vi "Testing Trigger.vi"() -> ()   [LabVIEW 2022 SP3]
panel:
  in  "2400 GPIB add":string="24"
  in  "2182 GPIB add":string="25"
  out "Delta Readings (uV)":ext[](array[numeric]) format="%.12f"
  out "Voltage Drop Across DUT":dbl[](graph)
  in  "Sample Count To Display":i32=10
  out "Resistance (m-Ohms)":dbl[](array[numeric]) format="%.10f"
  out "Resistance of DUT":dbl[](graph)
  in  "2400 Trig Count":string="20"
  in  "2182 Buffer Points":string="10"
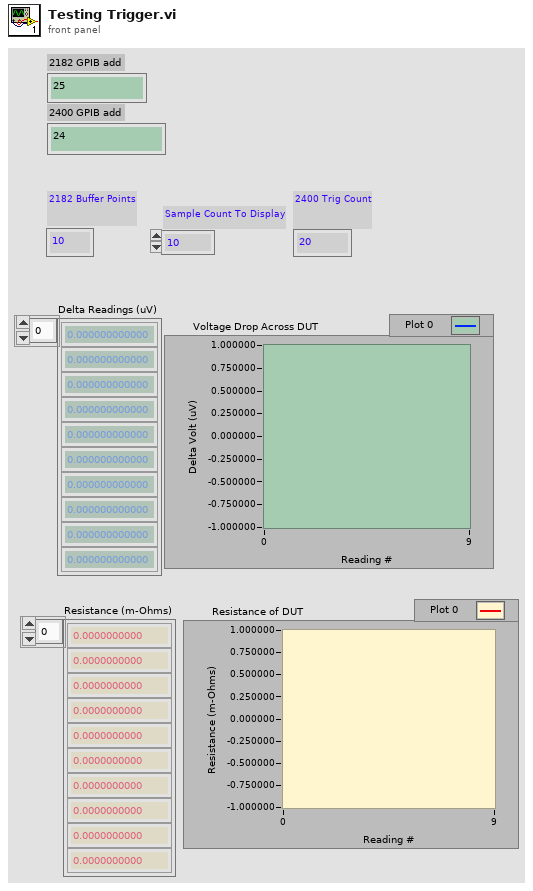
[diagram p1: front panel]
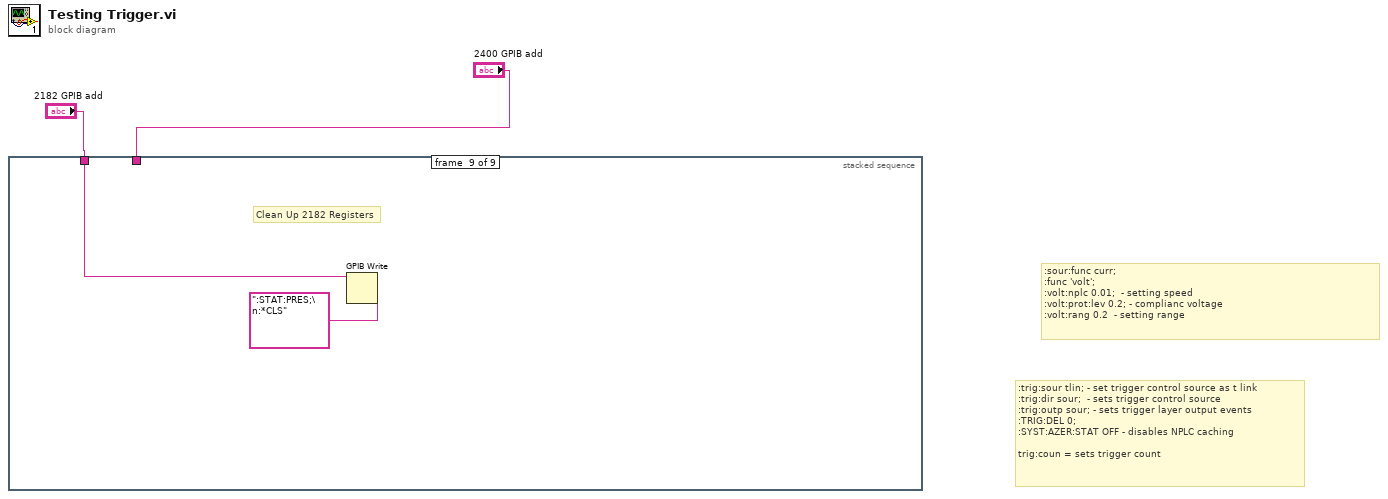
[diagram p0: block diagram]
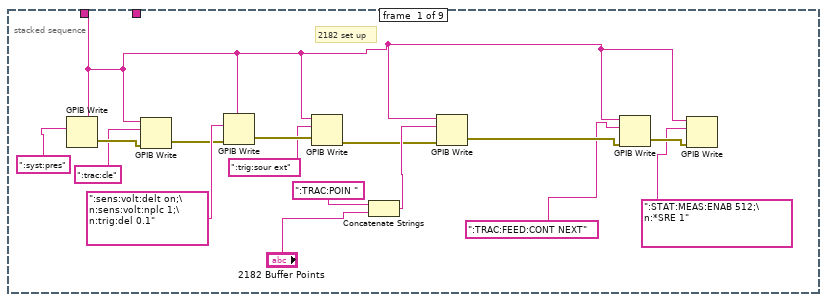
[diagram p2: hidden frame]
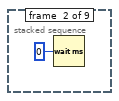
[diagram p3: hidden frame]
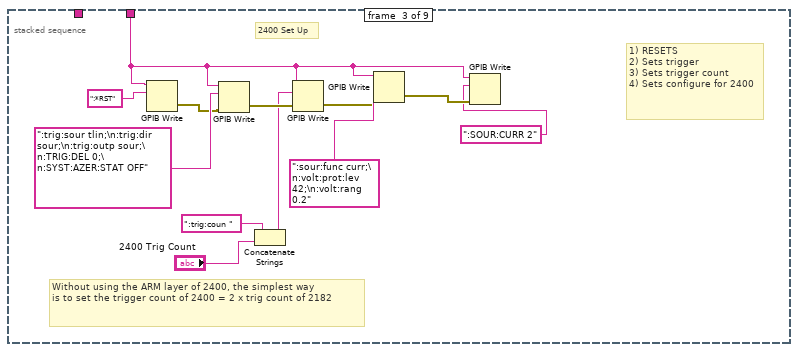
[diagram p4: hidden frame]
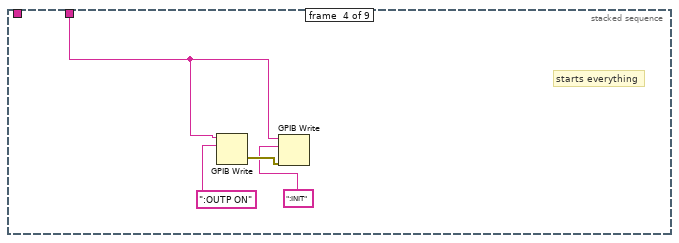
[diagram p5: hidden frame]
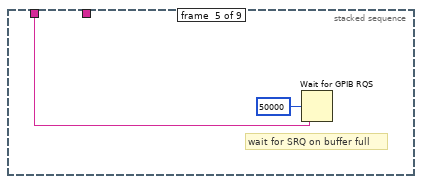
[diagram p6: hidden frame]
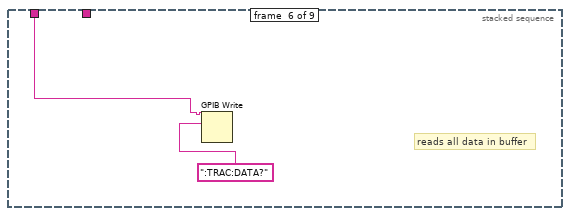
[diagram p7: hidden frame]
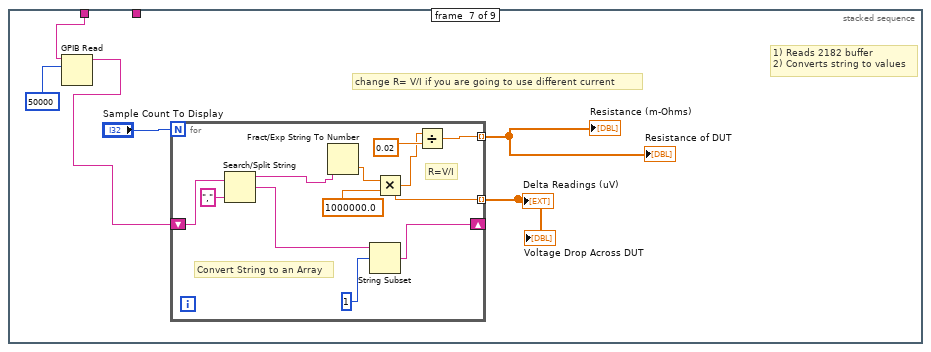
[diagram p8: hidden frame]
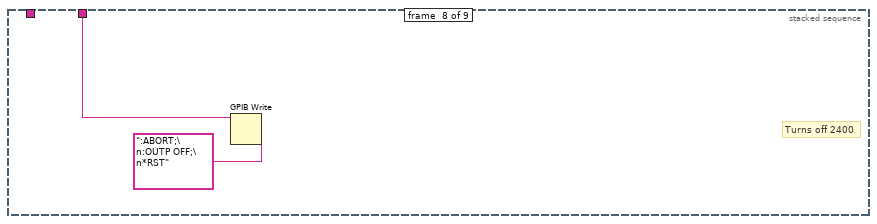
[diagram p9: hidden frame]
diagram:
  # ":trig:sour tlin; - set trigger control source as t link\n:trig:dir sour;  - sets trigger control source\n:trig:outp sour; - sets trigger layer output events\n:TRIG:DEL 0; \n:SYST:AZER:STAT OFF - disables NPLC caching              \n\ntrig:coun = sets trigger count"
  # ":sour:func curr;\n:func 'volt';\n:volt:nplc 0.01;  - setting speed\n:volt:prot:lev 0.2; - complianc voltage\n:volt:rang 0.2  - setting range"
  n1 = stacked-sequence {
    tunnel: "2182 GPIB add" -> [w6 _ _ _ w36 w38 w44 _ w59]
    tunnel: "2400 GPIB add" -> [_ _ w21 w32 _ _ _ w57 _]
    frame #0 {
      # "2182 set up"
      n2 = GPIB Write(0:w6, 1:":syst:pres") -> (6:w18:errorcluster)  [unwired: 3 in, 1 out]
      n3 = GPIB Write(0:w6, 1:":trac:cle", 3:w18) -> (6:w5:errorcluster)  [unwired: 2 in, 1 out]
      n4 = GPIB Write(0:w6, 1:":sens:volt:delt on;\n:sens:volt:nplc 1;\n:trig:del 0.1", 3:w5) -> (6:w9:errorcluster)  [unwired: 2 in, 1 out]
      n5 = GPIB Write(0:w6, 1:":trig:sour ext", 3:w9) -> (6:w4:errorcluster)  [unwired: 2 in, 1 out]
      n6 = Concatenate Strings(":TRAC:POIN ", "2182 Buffer Points") -> (w10:string)
      n7 = GPIB Write(0:w6, 1:w10, 3:w4) -> (6:w13:errorcluster)  [unwired: 2 in, 1 out]
      n8 = GPIB Write(0:w6, 1:":TRAC:FEED:CONT NEXT", 3:w13) -> (6:w15:errorcluster)  [unwired: 2 in, 1 out]
      n9 = GPIB Write(0:w6, 1:":STAT:MEAS:ENAB 512;\n:*SRE 1", 3:w15) -> ()  [unwired: 2 in, 2 out]
    }
    frame #1 {
      n10 = Wait (ms)(milliseconds to wait=u32 0) -> ()  [unwired: 1 out]
    }
    frame #2 {
      # "1) RESETS \n2) Sets trigger\n3) Sets trigger count\n4) Sets configure for 2400"
      # "Without using the ARM layer of 2400, the simplest way\nis to set the trigger count of 2400 = 2 x trig count of 2182"
      # "2400 Set Up"
      n11 = GPIB Write(0:w21, 1:":*RST") -> (6:w28:errorcluster)  [unwired: 3 in, 1 out]
      n12 = GPIB Write(0:w21, 1:":trig:sour tlin;\n:trig:dir sour;\n:trig:outp sour;\n:TRIG:DEL 0;\n:SYST:AZER:STAT OFF", 3:w28) -> (6:w27:errorcluster)  [unwired: 2 in, 1 out]
      n13 = Concatenate Strings(":trig:coun ", "2400 Trig Count") -> (w25:string)
      n14 = GPIB Write(0:w21, 1:w25, 3:w27) -> (6:w26:errorcluster)  [unwired: 2 in, 1 out]
      n15 = GPIB Write(0:w21, 1:":sour:func curr;\n:volt:prot:lev 42;\n:volt:rang 0.2", 3:w26) -> (6:w22:errorcluster)  [unwired: 2 in, 1 out]
      n16 = GPIB Write(0:w21, 1:":SOUR:CURR 2", 3:w22) -> ()  [unwired: 2 in, 2 out]
    }
    frame #3 {
      # "starts everything"
      n17 = GPIB Write(0:w32, 1:":OUTP ON") -> (6:w35:errorcluster)  [unwired: 3 in, 1 out]
      n18 = GPIB Write(0:w32, 1:":INIT", 3:w35) -> ()  [unwired: 2 in, 2 out]
    }
    frame #4 {
      # "wait for SRQ on buffer full"
      n19 = Wait for GPIB RQS(3:50000 ("timeout ms (488.2 global)"), 4:w36) -> ()  [unwired: 1 in, 2 out]
    }
    frame #5 {
      # "reads all data in buffer"
      n20 = GPIB Write(0:w38, 1:":TRAC:DATA?") -> ()  [unwired: 3 in, 2 out]
    }
    frame #6 {
      # "1) Reads 2182 buffer\n2) Converts string to values"
      # "change R= V/I if you are going to use different current"
      n21 = GPIB Read(0:w44, 1:50000 ("byte count")) -> (5:w42:string)  [unwired: 3 in, 2 out]
      n22 = for {
        N: "Sample Count To Display" -> [_]
        tunnel: [w47] -> w41 mode=indexing
        shift-right: [w52] -> _
        shift-left: w42 -> [w53]
        tunnel: [w49] -> w40 mode=indexing
        # "R=V/I"
        # "Convert String to an Array"
        n23 = Search/Split String(string=w53, search string/char (-)=",") -> (substring before match=w55:string, match + rest of string=w54:string)  [unwired: 1 in, 1 out]
        n24 = Fract/Exp String To Number(string=w55) -> (number=w46:dbl)  [unwired: 3 in, 1 out]
        n25 = String Subset(string=w54, offset (0)=1) -> (substring=w52:string)  [unwired: 1 in]
        n26 = Multiply(x=w46, y=1000000.0) -> (x*y=w47:dbl)
        n27 = Divide(x=w47, y=0.02 ("x")) -> (x/y=w49:dbl)
      }
      "Delta Readings (uV)" <- w41
      "Voltage Drop Across DUT" <- w41
      "Resistance (m-Ohms)" <- w40
      "Resistance of DUT" <- w40
    }
    frame #7 {
      # "Turns off 2400"
      n28 = GPIB Write(0:w57, 1:":ABORT;\n:OUTP OFF;\n*RST" ("data")) -> ()  [unwired: 3 in, 2 out]
    }
    frame #8 {
      # "Clean Up 2182 Registers"
      n29 = GPIB Write(0:w59, 1:":STAT:PRES;\n:*CLS" ("data")) -> ()  [unwired: 3 in, 2 out]
    }
  }
